vi "Record Maximum Values.vi"(5 "Reset":bool, 8 "Desired Iterations":u32=100, 9 "standard deviation (us)":dbl, 10 "jitter (us)":dbl) -> (0 "Stable?":bool, 1 "Stable Iterations":i32, 2 "Max Std Dev (us)":dbl, 3 "Max Jitter (us)":dbl)   [LabVIEW 2014]
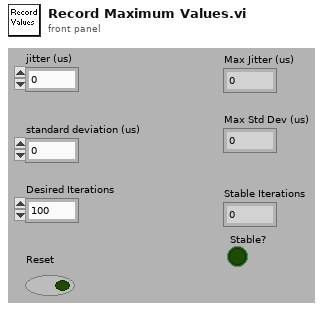
[diagram p1: front panel]
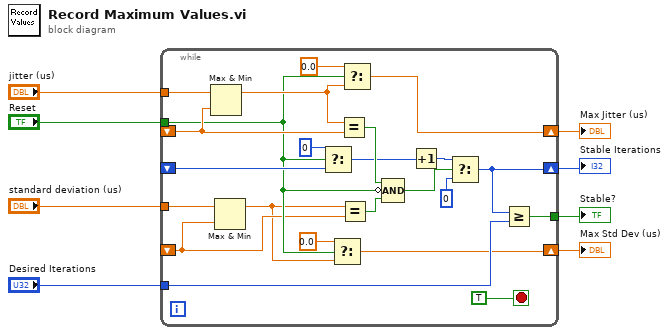
[diagram p0: block diagram]
diagram:
  n1 = while {
    shift-right: [w9] -> w3
    shift-left: _ -> [w11]
    shift-right: [w15] -> w4
    shift-left: _ -> [w18]
    tunnel: "standard deviation (us)" -> [w29]
    tunnel: "jitter (us)" -> [w28]
    shift-right: [w26] -> w2
    shift-left: _ -> [w22]
    tunnel: [w24] -> w6
    tunnel: "Desired Iterations" -> [w19]
    tunnel: "Reset" -> [w12]
    stop <- TRUE stop-if-true
    n2 = Max & Min(x=w28, y=w18) -> (max(x,y)=w16:dbl)  [unwired: 1 out]
    n3 = Max & Min(x=w29, y=w11) -> (max(x,y)=w10:dbl)  [unwired: 1 out]
    n4 = Select(t=0, s=w12, f=w22) -> (s? t:f=w20:i32)
    n5 = Select(t=0.0, s=w12, f=w10) -> (s? t:f=w9:dbl)
    n6 = Equal?(x=w16, y=w18) -> (x = y?=w27:bool)
    n7 = Equal?(x=w10, y=w11) -> (x = y?=w14:bool)
    n8 = Select(t=0.0, s=w12, f=w16) -> (s? t:f=w15:dbl)
    n9 = Compound Arithmetic op=AND(w27, invert w12, w14) -> (w25:bool)
    n10 = Increment(x=w20) -> (x+1=w30:i32)
    n11 = Select(t=w30, s=w25, f=0) -> (s? t:f=w26:i32)
    n12 = Greater Or Equal?(x=w26, y=w19) -> (x >= y?=w24:bool)
  }
  "Stable?" <- w6
  "Max Jitter (us)" <- w4
  "Max Std Dev (us)" <- w3
  "Stable Iterations" <- w2
